vi "Check Versions.vi"(0 "Register Buses":refnum<class "ni579x Register Bus v1 Host.lvclass">[](array[class]), 11 "error in":errorcluster) -> (4 "Register Buses (out)":refnum<class "ni579x Register Bus v1 Host.lvclass">[](array[class]), 15 "error out":errorcluster)   [LabVIEW 2012, in "ni579x Synchronization v1 Host.lvlib"]
uses:
  <instrlib>/ni579x/Synchronization/v1/Host/ni579x Synchronization v1 Host.lvlib
  <instrlib>/ni579x/Register Bus/v1/Host/ni579x Register Bus v1 Host.lvclass
  <instrlib>/ni579x/Register Bus/v1/Host/Public/Register Read Request.ctl
  <instrlib>/ni579x/Synchronization/v1/Shared/ni579x Synchronization Register Addresses.ctl
  <instrlib>/ni579x/Config/v1/Shared/Types/ni579x Register Bus Subsystem ID.ctl
  <vilib>/Utility/error.llb/Error Cluster From Error Code.vi
  <vilib>/ErrorRing/Error Ring.xnode
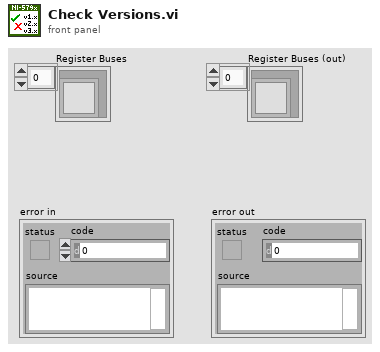
[diagram p1: front panel]
types:
  T1 = typedef "ni579x Register Bus Subsystem ID.ctl" = u8
  T2 = typedef "ni579x Synchronization Register Addresses.ctl" = enum16{"Signature", "Current Version", "Oldest Compatible Version", "Scratch Register", "sync.master", "sync.meas.enable", "sync.meas.ready", "sync.meas.arm", "sync.meas.valid", "sync.meas.value", "sync.cptr.adjust", "sync.cptr.period", "sync.meas.oversample factor"}
  T3 = typedef "ni579x Register Bus v1 Host.lvclass/Register Read Request.ctl" = cluster{"subsystem":u8, "address":u16}
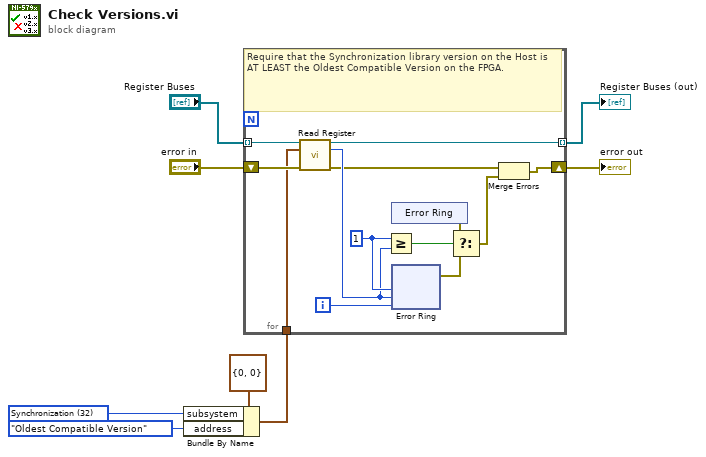
[diagram p0: block diagram]
diagram:
  w6 = T1 32 items=["FAM Register Operation"=0, "User Command"=16, "Synchronization"=32] ("Subsystem ID")
  n1 = Bundle By Name(cluster=T3 {"subsystem"=0, "address"=0} ("register read request"), "subsystem"=w6, "address"=ni579x_Synchronization_Register_Addresses."Oldest Compatible Version" ("Synchronization Registers")) -> (w8:T3)
  n2 = for {
    tunnel: "Register Buses" -> [w20] mode=indexing
    shift-right: [w11] -> w4
    shift-left: "error in" -> [w21]
    tunnel: w8 -> [w19]
    tunnel: [w10] -> w3 mode=indexing
    i -> [w13]
    w15 = u32 1 ("data")
    # "Require that the Synchronization library version on the Host is AT LEAST the Oldest Compatible Version on the FPGA."
    n3 = call <instrlib>:"Read Register.vi"("session in"=w20, "register read request"=w19, "error in"=w21) -> ("session out"=w10:refnum<class "ni579x Register Bus v1 Host.lvclass">, "data"=w14:u32, "error out"=w12:errorcluster)  [unwired: 10 in]
    n4 = Greater Or Equal?(x=w15, y=w14) -> (x >= y?=w9:bool)
    n5 = xnode "Error Ring"() -> ("error out"=w16:errorcluster)
    n6 = xnode "Error Ring"("parameter 0"=w15, "parameter 1"=w14, "parameter 2"=w13) -> ("error out"=w18:errorcluster)
    n7 = Select(t=w16, s=w9, f=w18) -> (s? t:f=w17:errorcluster)
    n8 = Merge Errors(w12, w17) -> (w11:errorcluster)
  }
  "error out" <- w4
  "Register Buses (out)" <- w3
